vi "ArmPathPlanner.vi"(0 "StartPoint":T5, 1 "EndPoint":T5, 2 "PathPointSpacing (in)":dbl=0.25, 3 "MinArmLength":dbl=44.0, 4 "MaxArmLength":dbl=68.0, 5 "AvoidancePolygon":T4, 7 "MotionProfileGeneratorParameters":T3={"Trajectory Point Interval (ms)"=10, "Maximum Travel Speed (units/s)"=0.0, "Velocity Ramp Time (ms)"=0.0, "Acceleration Ramp Time (ms)"=1.0} {"Acceleration Ramp Time (ms)" min=1.0; "Velocity Ramp Time (ms)" min=1.0; "Maximum Travel Speed (units/s)" min=0.0; "Trajectory Point Interval (ms)" items=["TrajectoryDuration_0ms"=0, "TrajectoryDuration_5ms"=5, "TrajectoryDuration_10ms"=10, "TrajectoryDuration_20ms"=20, "TrajectoryDuration_30ms"=30, "TrajectoryDuration_40ms"=40, "TrajectoryDuration_50ms"=50, "TrajectoryDuration_100ms"=100]}) -> (14 "Path":T6[](array[typedef]), 15 "ShoulderPath":T1[](array[typedef]) {"Time (ms)" items=["TrajectoryDuration_0ms"=0, "TrajectoryDuration_5ms"=5, "TrajectoryDuration_10ms"=10, "TrajectoryDuration_20ms"=20, "TrajectoryDuration_30ms"=30, "TrajectoryDuration_40ms"=40, "TrajectoryDuration_50ms"=50, "TrajectoryDuration_100ms"=100]}, 16 "ExtendPath":T1[](array[typedef]) {"Time (ms)" items=["TrajectoryDuration_0ms"=0, "TrajectoryDuration_5ms"=5, "TrajectoryDuration_10ms"=10, "TrajectoryDuration_20ms"=20, "TrajectoryDuration_30ms"=30, "TrajectoryDuration_40ms"=40, "TrajectoryDuration_50ms"=50, "TrajectoryDuration_100ms"=100]}, 17 "WristPath":T1[](array[typedef]) {"Time (ms)" items=["TrajectoryDuration_0ms"=0, "TrajectoryDuration_5ms"=5, "TrajectoryDuration_10ms"=10, "TrajectoryDuration_20ms"=20, "TrajectoryDuration_30ms"=30, "TrajectoryDuration_40ms"=40, "TrajectoryDuration_50ms"=50, "TrajectoryDuration_100ms"=100]}, 19 "PathLength (in)":dbl)   [LabVIEW 2018]
uses:
  TypeDefs/ArmCoordinate.ctl
  ArgosLib/Path Planning/TypeDefs/Point2D.ctl
  ArgosLib/Path Planning/TypeDefs/Polygon2D.ctl
  General/MotionProfiling/TypeDefs/MotionProfileGeneratorParams.ctl
  <vilib>/Rock Robotics/WPI/ThirdParty/Phoenix-LabVIEW/Motor Controller/Controls/CTRE_Phoenix_MotorControl_TrajectoryPointTimeDur.ctl
  General/MotionProfiling/TypeDefs/TrajectoryPoint.ctl
  ArgosLib/ArgosLib.lvlib
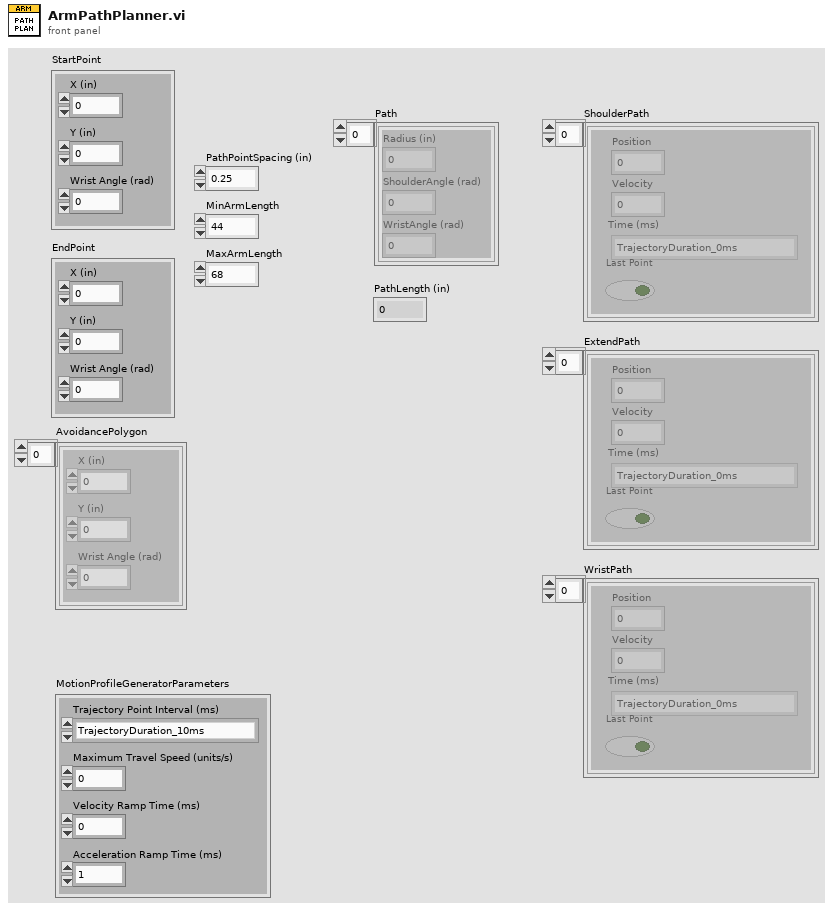
[diagram p1: front panel]
types:
  T1 = typedef "TrajectoryPoint.ctl" = cluster{"Position ":dbl, "Velocity ":dbl, "Time (ms)":T2, "Last Point":bool}
  T2 = typedef "CTRE_Phoenix_MotorControl_TrajectoryPointTimeDur.ctl" = i32
  T3 = typedef "MotionProfileGeneratorParams.ctl" = cluster{"Trajectory Point Interval (ms)":T2, "Maximum Travel Speed (units/s)":dbl, "Velocity Ramp Time (ms)":dbl, "Acceleration Ramp Time (ms)":dbl}
  T4 = typedef "ArgosLib.lvlib/Polygon2D.ctl" = T5[]
  T5 = typedef "ArgosLib.lvlib/Point2D.ctl" = cluster{"X (in)":dbl, "Y (in)":dbl, "Wrist Angle (rad)":dbl}
  T6 = typedef "ArmCoordinate.ctl" = cluster{"Radius (in)":dbl, "ShoulderAngle (rad)":dbl, "WristAngle (rad)":dbl}
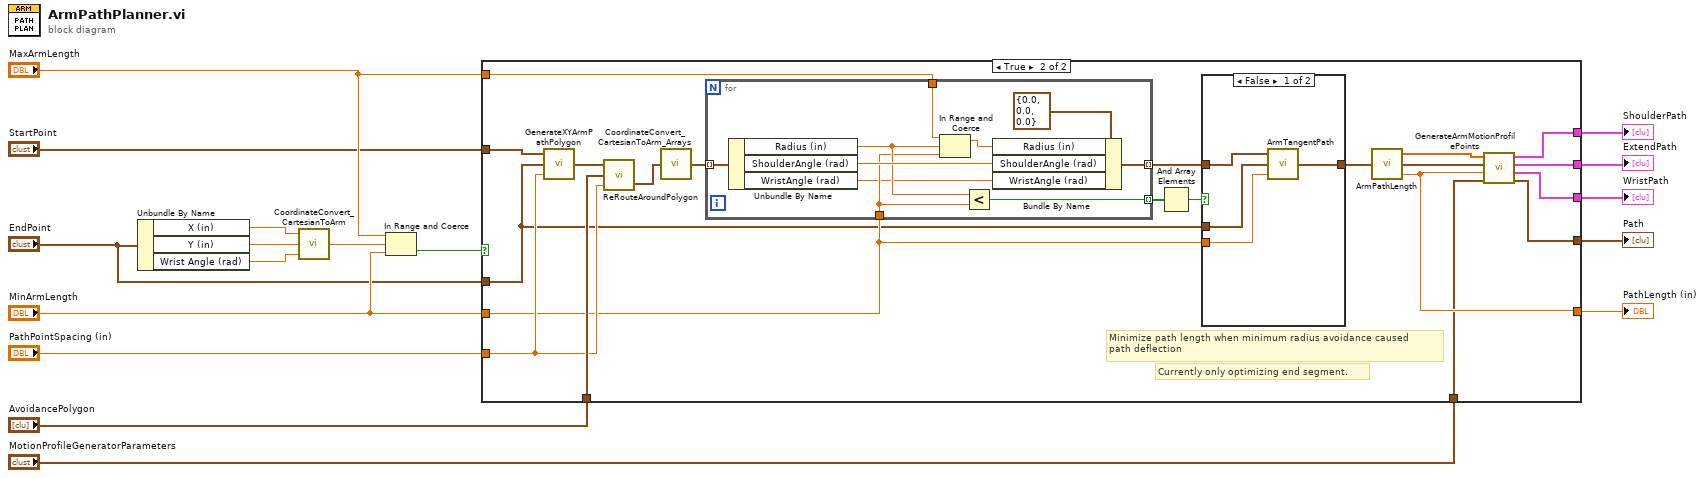
[diagram p0: block diagram]
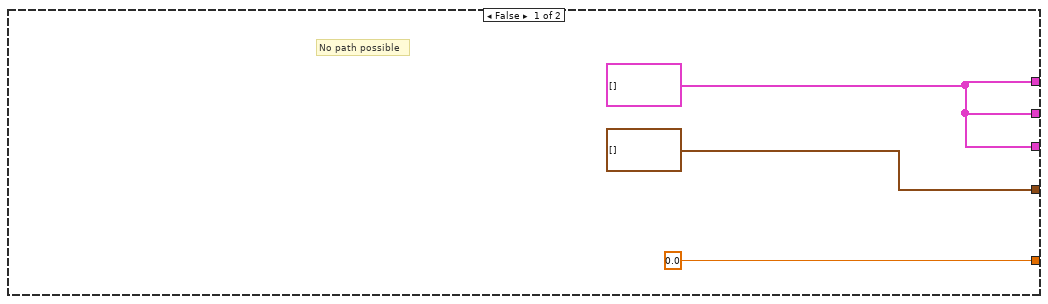
[diagram p2: hidden frame]
diagram:
  n1 = Unbundle By Name("EndPoint") -> ("X (in)"=w10:dbl, "Y (in)"=w9:dbl, "Wrist Angle (rad)"=w1:dbl)
  n2 = call "CoordinateConvert_CartesianToArm.vi"("Wrist (rad)"=w1, "Y (in)"=w9, "X (in)"=w10) -> ("Radius (in)"=w17:dbl)  [unwired: 2 out]
  n3 = In Range and Coerce(upper limit="MaxArmLength", x=w17, lower limit="MinArmLength") -> (In Range?=w16:bool)  [unwired: 1 out]
  n4 = case shown="True" w16 {
    tunnel: [T6[] [] ("ArmPathOut") w30] -> w11
    tunnel: [0.0 w32] -> w15
    tunnel: "MinArmLength" -> [_ w23]
    tunnel: "MaxArmLength" -> [_ w41]
    tunnel: "PathPointSpacing (in)" -> [_ w36]
    tunnel: "StartPoint" -> [_ w40]
    tunnel: "EndPoint" -> [_ w22]
    tunnel: "AvoidancePolygon" -> [_ w37]
    tunnel: "MotionProfileGeneratorParameters" -> [_ w31]
    tunnel: [w18 w29] -> w4
    tunnel: [w18 w28] -> w3
    tunnel: [w18 w21] -> w2
    frame False {
      w18 = T1[] [] ("ExtendPath")
      # "No path possible"
    }
    frame True {
      # "Currently only optimizing end segment."
      # "Minimize path length when minimum radius avoidance caused\npath deflection"
      n5 = call "GenerateXYArmPathPolygon.vi"("PointSpacing (in)"=w36, "EndPoint"=w22, "StartPoint"=w40) -> ("XYPathPoints"=w38:T5[])
      n6 = call "ReRouteAroundPolygon.vi"("Desired Point Spacing (in)"=w36, "AvoidancePolygon"=w37, "InputPath"=w38) -> ("OutputPath"=w35:T5[])  [unwired: 1 out]
      n7 = call "CoordinateConvert_CartesianToArm_Arrays.vi"("XYPoints"=w35) -> ("ArmCoordinates"=w39:T6[])
      n8 = for {
        tunnel: w41 -> [w56]
        tunnel: w23 -> [w49]
        tunnel: w39 -> [w55] mode=indexing
        tunnel: [w51] -> w25 mode=indexing
        tunnel: [w48] -> w27 mode=indexing
        n9 = Unbundle By Name(w55) -> ("Radius (in)"=w50:dbl, "ShoulderAngle (rad)"=w54:dbl, "WristAngle (rad)"=w47:dbl)
        n10 = In Range and Coerce(upper limit=w56, x=w50, lower limit=w49) -> (coerced(x)=w53:dbl)  [unwired: 1 out]
        n11 = Less?(x=w50, y=w49) -> (x < y?=w48:bool)
        n12 = Bundle By Name(cluster=T6 {"Radius (in)"=0.0, "ShoulderAngle (rad)"=0.0, "WristAngle (rad)"=0.0} ("Point"), "Radius (in)"=w53, "ShoulderAngle (rad)"=w54, "WristAngle (rad)"=w47) -> (w51:T6)
      }
      n13 = And Array Elements(Boolean array=w27) -> (logical AND=w26:bool)
      n14 = case shown="False" w26 {
        tunnel: w25 -> [w45 w46]
        tunnel: [w42 w46] -> w24
        tunnel: w23 -> [w43 _]
        tunnel: w22 -> [w44 _]
        frame False {
          n15 = call "ArmTangentPath.vi"("Radius"=w43, "EndPoint"=w44, "PathIn"=w45) -> ("PathOut"=w42:T6[])
        }
        frame True {
        }
      }
      n16 = call "ArmPathLength.vi"("ArmPathIn"=w24) -> ("Path Length"=w32:dbl, "ArmPathOut"=w33:T6[], "IndexedPathLength"=w34:dbl[])  [unwired: 2 in]
      n17 = call "GenerateArmMotionProfilePoints.vi"("MotionProfileGeneratorParameters"=w31, "PathDistance"=w32, "ArmPathIn"=w33, "IndexedPathLength"=w34) -> ("ArmPathOut"=w30:T6[], "WristPath"=w21:T1[], "ExtendPath"=w28:T1[], "ShoulderPath"=w29:T1[])
    }
  }
  "PathLength (in)" <- w15
  "Path" <- w11
  "ShoulderPath" <- w4
  "ExtendPath" <- w3
  "WristPath" <- w2
